vi "seed_analysis.vi"() -> ()   [LabVIEW 2023]
uses:
  <vilib>/vision/NI_Vision_Development_Module.lvlib
panel:
  out "数值 2":i32
  out "Y":dbl
  out "X":dbl
  out "Center of Mass":cluster{"X":dbl, "Y":dbl}
  out "数值":i32
  out "Orientation":dbl
  out "Threshold Image":T1(plugin-control)
  out "Selected Particle Report":T2 {"Orientation" format="%.2f"; "Center of Mass"."Y" format="%.2f"; "Center of Mass"."X" format="%.2f"}
  in  "Stop":bool
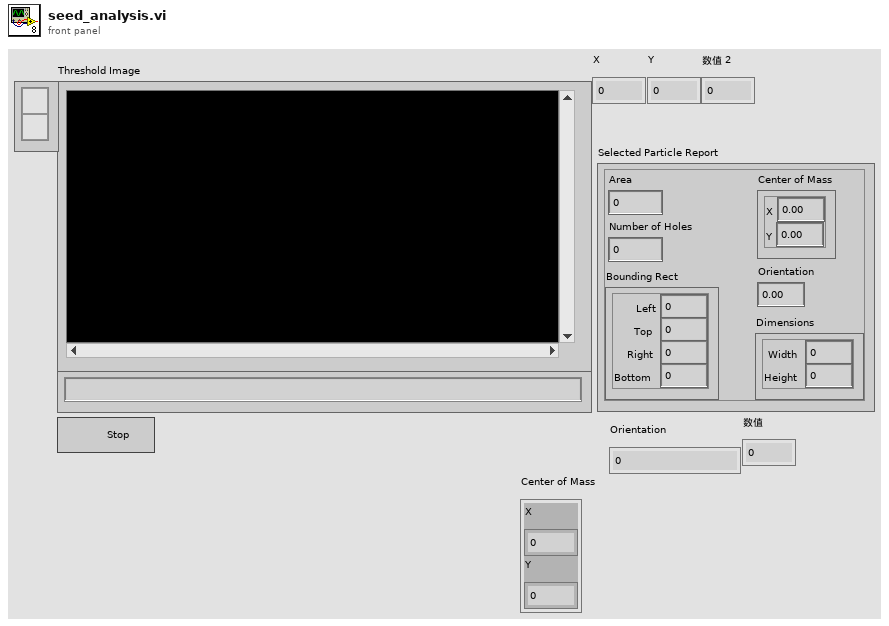
[diagram p1: front panel]
types:
  T1 = typedef "IMAQ Image.ctl" = refnum<image>
  T2 = cluster{"Area":dbl, "Number of Holes":dbl, "Bounding Rect":cluster{"Left":dbl, "Top":dbl, "Right":dbl, "Bottom":dbl}, "Center of Mass":cluster{"X":dbl, "Y":dbl}, "Orientation":dbl, "Dimensions":cluster{"Width":dbl, "Height":dbl}}
  T3 = cluster{"Area":dbl, "Number of Holes":dbl, "Bounding Rect":cluster{"Left":dbl, "Top":dbl, "Right":dbl, "Bottom":dbl}, "Center of Mass":cluster{"X":dbl, "Y":dbl}, "Orientation":dbl, "Dimensions":cluster{"Width":dbl, "Height":dbl}}[]
  T4 = cluster{"Left":dbl, "Top":dbl, "Right":dbl, "Bottom":dbl}
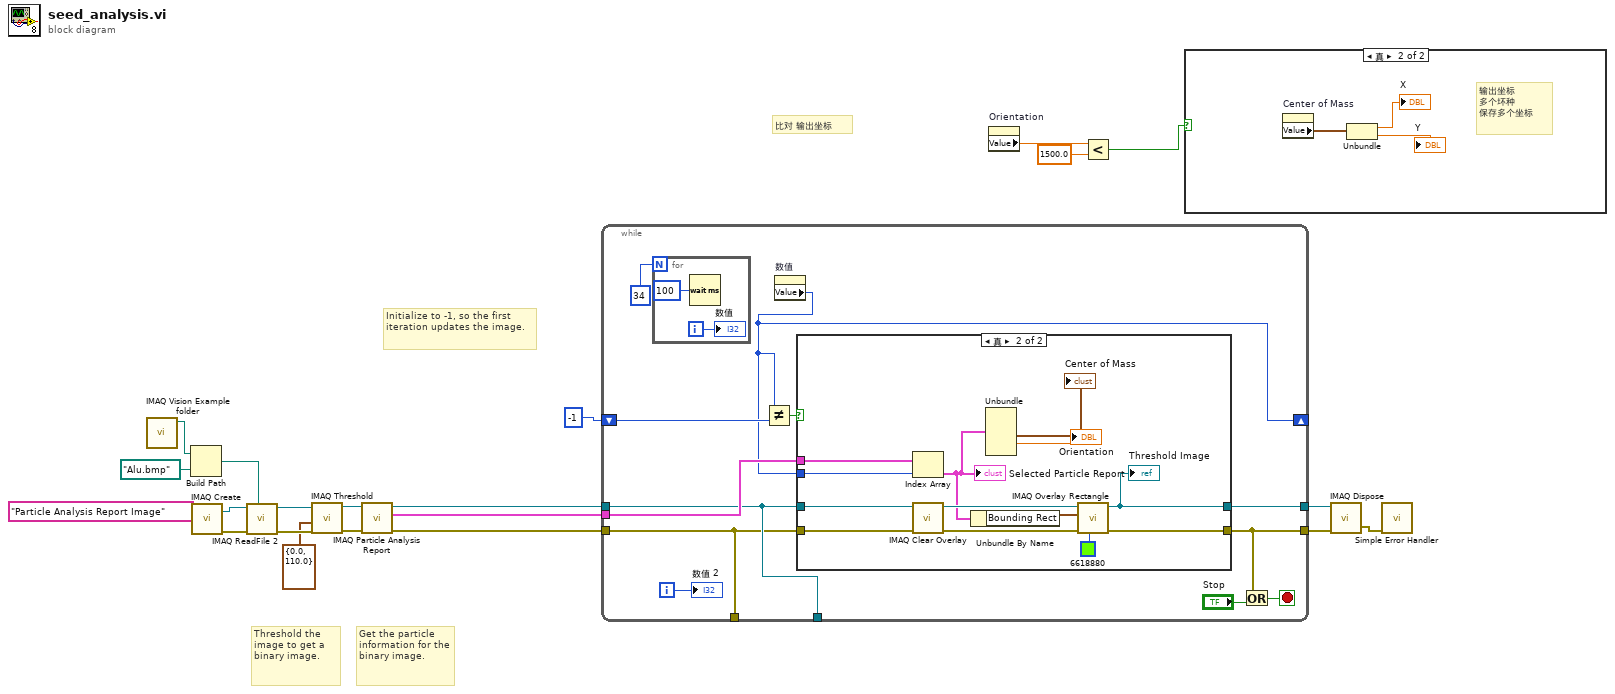
[diagram p0: block diagram]
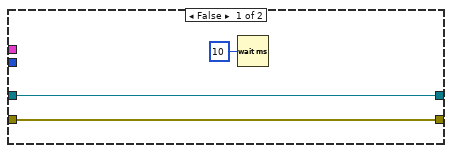
[diagram p3: hidden frame]
diagram:
  # "比对 输出坐标"
  # "Initialize to -1, so the first iteration updates the image."
  # "Get the particle information for the binary image."
  # "Threshold the image to get a binary image."
  n1 = call "IMAQ Vision Example folder.vi"() -> ("Example Image Path"=w18:path)  [unwired: 11 in]
  n2 = Build Path(base path=w18, name or relative path=path "Alu.bmp") -> (appended path=w16:path)
  n3 = call "IMAQ Create"("Image Name"="Particle Analysis Report Image") -> ("New Image"=w20:T1, "error out"=w19:errorcluster)  [unwired: 4 in]
  n4 = call "IMAQ ReadFile 2"("File Path"=w16, "error in (no error)"=w19, "Image"=w20) -> ("error out"=w14:errorcluster, "Image Out"=w15:T1)  [unwired: 4 in, 3 out]
  n5 = call "IMAQ Threshold"("error in (no error)"=w14, "Range"=cluster{"Lower value":sgl, "Upper value":sgl} {"Lower value"=0.0, "Upper value"=110.0}, "Image Src"=w15) -> ("error out"=w13:errorcluster, "Image Dst Out"=w12:T1)  [unwired: 7 in]
  n6 = call "IMAQ Particle Analysis Report"("error in (no error)"=w13, "Image"=w12) -> ("error out"=w9:errorcluster, "Particle Reports (Pixels)"=w4:T3, "Image Out (duplicate)"=w10:T1)  [unwired: 4 in, 3 out]
  n7 = while {
    tunnel: w10 -> [w26]
    tunnel: w9 -> [w25]
    tunnel: [w28] -> w8
    tunnel: [w33] -> w7
    tunnel: w4 -> [w31]
    shift-right: [w24] -> _
    shift-left: -1 ("Selected Particle") -> [w32]
    tunnel: [w26] -> _
    tunnel: [w25] -> _
    i -> [w22]
    stop <- w27 stop-if-true
    n8 = for {
      N: 34 -> [_]
      i -> [w35]
      n9 = Wait (ms)(milliseconds to wait=u32 100 ("等待时间（毫秒）")) -> ()  [unwired: 1 out]
      "数值" <- w35
    }
    n10 = property on="数值" class="DigNum (严格)"() -> ("Value"=w24:i32)  [unwired: 2 in, 2 out]
    n11 = Not Equal?(x=w24, y=w32) -> (x != y?=w30:bool)
    n12 = case shown="真" w30 {
      tunnel: w26 -> [w38 w47]
      tunnel: w25 -> [w37 w46]
      tunnel: [w37 w51] -> w28
      tunnel: [w38 w43] -> w33
      tunnel: w31 -> [_ w48]
      tunnel: w24 -> [_ w42]
      frame False {
        n13 = Wait (ms)(milliseconds to wait=u32 10) -> ()  [unwired: 1 out]
      }
      frame True {
        n14 = Index Array(array=w48, index=w42) -> (element=w41:T2)
        "Selected Particle Report" <- w41
        n15 = call "IMAQ Clear Overlay"("error in (no error)"=w46, "Image"=w47) -> ("error out"=w44:errorcluster, "Image Out"=w45:T1)  [unwired: 8 in]
        n16 = Unbundle By Name(w41) -> ("Bounding Rect"=w50:T4)
        n17 = Unbundle(w41) -> ("Center of Mass"=→"Center of Mass":cluster{"X":dbl, "Y":dbl}, "Orientation"=→"Orientation":dbl)  [unwired: 4 out]
        n18 = call "IMAQ Overlay Rectangle"("Color"=u32 6618880, "error in (no error)"=w44, "Rectangle"=w50, "Image"=w45) -> ("error out"=w51:errorcluster, "Image Out"=w43:T1)  [unwired: 6 in]
        "Threshold Image" <- w43
      }
    }
    n19 = Or(x=w28, y="Stop") -> (x .or. y?=w27:bool)
    "数值 2" <- w22
  }
  n20 = property on="Orientation" class="DigNum (严格)"() -> ("Value"=w3:dbl)  [unwired: 2 in, 2 out]
  n21 = Less?(x=w3, y=1500.0) -> (x < y?=w1:bool)
  n22 = case shown="真" w1 {
    frame False {
    }
    frame True {
      # "输出坐标\n多个坏种\n保存多个坐标"
      n23 = property on="Center of Mass" class="Clust (严格)"() -> ("Value"=w54:cluster{"X":dbl, "Y":dbl})  [unwired: 2 in, 2 out]
      n24 = Unbundle(w54) -> ("X"=→"X":dbl, "Y"=→"Y":dbl)
    }
  }
  n25 = call "IMAQ Dispose"("Image"=w7, "error in (no error)"=w8) -> ("error out"=w11:errorcluster)  [unwired: 4 in]
  n26 = call <vilib>:"Simple Error Handler.vi"("error in (no error)"=w11) -> ()  [unwired: 4 in, 5 out]
